vi "Advance past pure whitespace.vi"(7 "JSON":string, 9 "Offset":i32) -> (1 "Offset of first non-whitespace":i32, 3 "Parser State":T1)   [LabVIEW 2020, in "JSONtext.lvlib"]
uses:
  <vilib>/JDP Science/JSONtext/JSONtext.lvlib
  <vilib>/JDP Science/JSONtext/Parsing/Parsing State.ctl
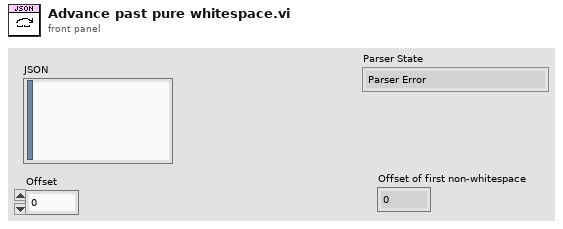
[diagram p1: front panel]
types:
  T1 = typedef "JSONtext.lvlib/Parsing State.ctl" = enum16{"Parser Error", "Object", "Array", "String", "Number/Other", "Leading Whitespace", "Object end", "Array end", "Value end"}
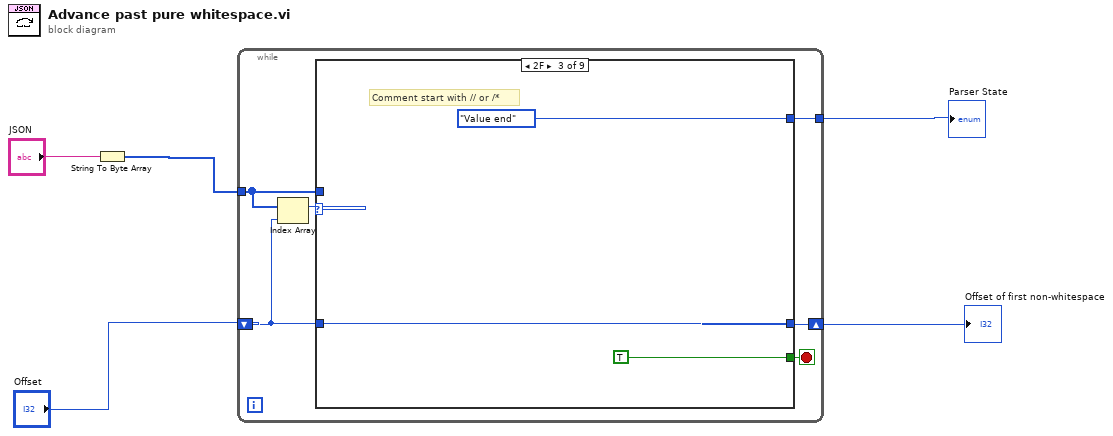
[diagram p0: block diagram]
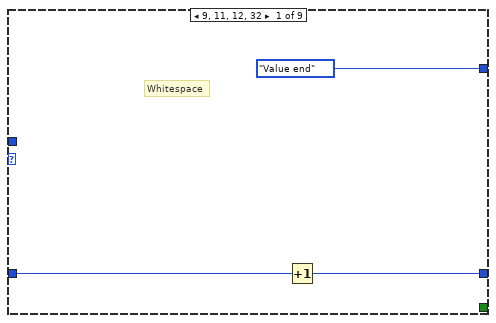
[diagram p2: hidden frame]
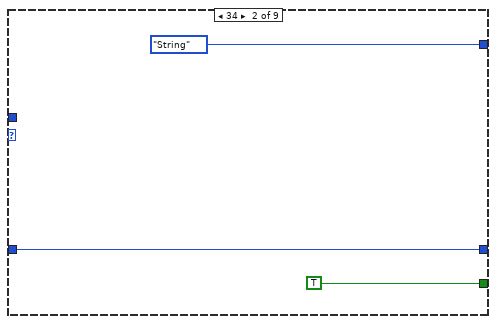
[diagram p3: hidden frame]
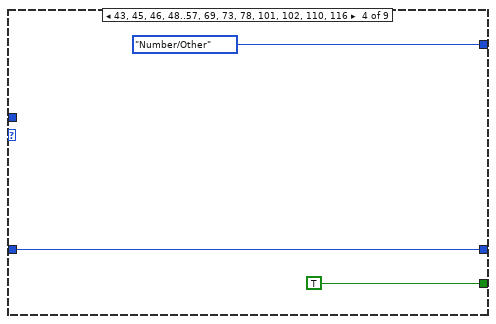
[diagram p4: hidden frame]
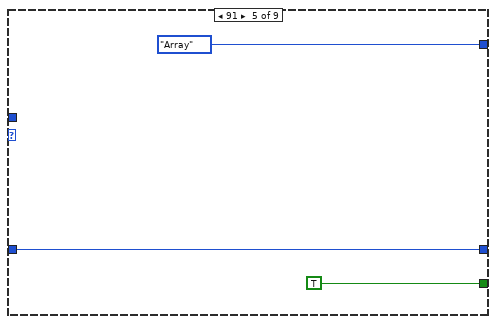
[diagram p5: hidden frame]
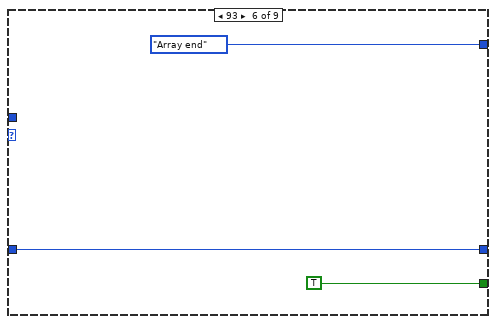
[diagram p6: hidden frame]
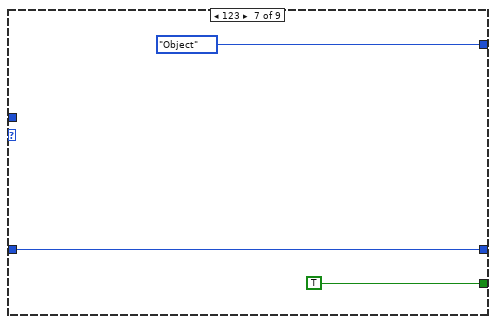
[diagram p7: hidden frame]
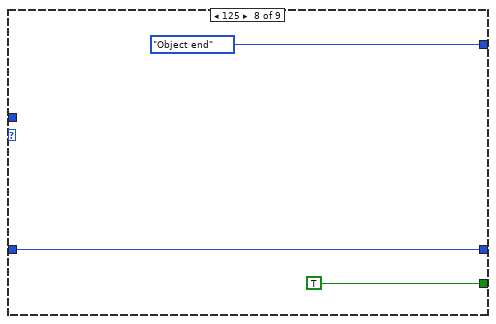
[diagram p8: hidden frame]
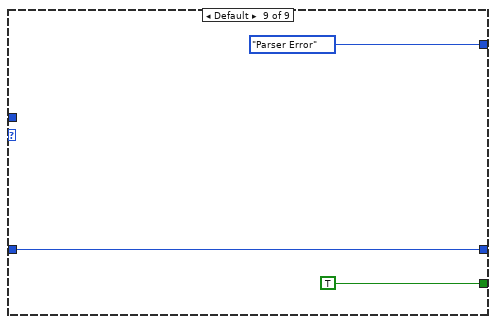
[diagram p9: hidden frame]
diagram:
  n1 = String To Byte Array(string="JSON") -> (unsigned byte array=w2:u8[])
  n2 = while {
    tunnel: w2 -> [w6]
    shift-right: [w7] -> w4
    shift-left: "Offset" -> [w8]
    tunnel: [w10] -> w5
    stop <- w9 stop-if-true
    n3 = Index Array(array=w6, index=w8) -> (element=w11:u8)
    n4 = case shown="2F" w11 {
      tunnel: [Parsing_State."Value end" Parsing_State."String" Parsing_State."Value end" Parsing_State."Number/Other" Parsing_State."Array" Parsing_State."Array end" Parsing_State."Object" Parsing_State."Object end" Parsing_State."Parser Error"] -> w10
      tunnel: [_ TRUE TRUE TRUE TRUE TRUE TRUE TRUE TRUE] -> w9
      tunnel: w8 -> [w14 w15 w18 w21 w24 w27 w30 w33 w38]
      tunnel: [w13 w15 w18 w21 w24 w27 w30 w33 w38] -> w7
      tunnel: w6 -> [_ _ _ _ _ _ _ _ _]
      frame 9, 11, 12, 32 {
        # "Whitespace"
        n5 = Increment(x=w14) -> (x+1=w13:i32)
      }
      frame 34 {
      }
      frame 47 {
        # "Comment start with // or /*"
      }
      frame 43, 45, 46, 48..57, 69, 73, 78, 101, 102, 110, 116 {
      }
      frame 91 {
      }
      frame 93 {
      }
      frame 123 {
      }
      frame 125 {
      }
      frame Default {
      }
    }
  }
  "Parser State" <- w5
  "Offset of first non-whitespace" <- w4
